vi "Reply.vi"(4 "Is Priority":bool, 6 "Sender":refnum<class "Sender.lvclass">, 7 "Actor in":refnum<class "Actor.lvclass">, 9 "Error":errorcluster, 10 "Actor":refnum<class "Actor.lvclass">) -> (0 "Error out":errorcluster)   [LabVIEW 2025, in "jettl.lvlib" / "Finish Msg.lvlib"]
uses:
  Finish Msg.lvlib
  Finish Msg/Finish Msg.lvclass
  C:/git/jettl/src/jettl/jettl/Finish Msg/Finish Msg/Finish Msg.lvclass
  C:/git/jettl/src/jettl/jettl/Msg/Msg.lvclass
  Actor/Actor/Actor.lvclass
  Sender/Sender/Sender.lvclass
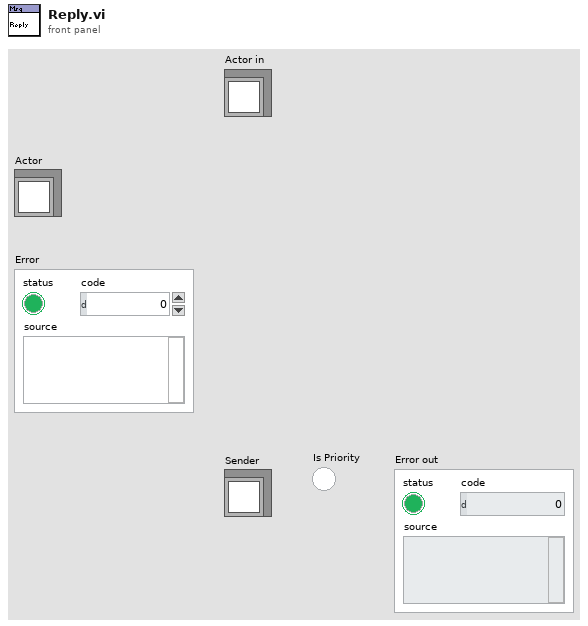
[diagram p1: front panel]
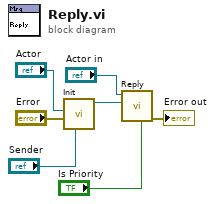
[diagram p0: block diagram]
diagram:
  n1 = call "Init.vi"("Sender"="Sender", "Error"="Error", "Actor"="Actor") -> ("Finish Msg out"=w3:refnum<class "Finish Msg.lvclass">)  [unwired: 8 in]
  n2 = call-dynamic "Reply.vi"("Is Priority"="Is Priority", "Msg"=w3, "Actor in"="Actor in") -> ("Error out"=→"Error out":errorcluster)  [unwired: 8 in]
